vi "Digital Pattern Generation.vi"() -> ()   [LabVIEW 2020]
doc: "This example demonstrates how to acquire a continuous amount of digital data based off of a sample clock.\n\nSome hardware (e.g. M Series DAQ) must use an external sample clock for digital tasks. To view a complete list of available sample clock sources, consult the Device Routes table in Measurement and Automation Explorer.\n\nFor instructions on how to connect your signals to the DAQ device, refer to your device documentation."
uses:
  <vilib>/Utility/error.llb/DialogType.ctl
  <vilib>/DAQmx/read.llb/DAQmx Read (Digital Wfm 1Chan NSamp).vi
  <vilib>/DAQmx/create/channels.llb/DAQmx Create Channel (DI-Digital Input).vi
  <vilib>/Utility/file.llb/Read Delimited Spreadsheet (DBL).vi
  <vilib>/DAQmx/configure/timing.llb/DAQmx Timing (Sample Clock).vi
  <vilib>/DAQmx/miscellaneous.llb/DAQmx Fill In Error Info.vi
  <vilib>/Waveform/DWDTOps.llb/DWDT Digital to Analog.vi
  <vilib>/Analysis/polynomials.llb/Unique Numbers and Multiplicity (DBL).vi
  <vilib>/Analysis/NI_AALPro.lvlib
panel:
  in  "Crank or Cam":enum16{"Crank", "Cam"}(ring)
  out "Pass?":bool=TRUE
  out "Waveform Graph 2":waveform(dbl)(graph)={"t0"=timestamp(0 s since 1904-01-01), "dt"=0.0001, "Y"=array[40000 elements]}
  out "indices of samples equal to 1":i32[](array[numeric])
  out "number of samples equal to 1":i32=6448
  out "number of samples in each valley":i32[](array[numeric])=[140, 139, 140, 140, 140, 140, 140, 140, 140, 140, 139, 140, 140, 139, 140, 140, 139, 140, 140, 140, 140, 140, 140, 140, 140, 139, 140, 140, 139, 140, 140, 140, 140, 473, 140, 140, 140, 140, 139, 140, 140, 140, 140, 140, 140, 140, 140, 140, 140, 140, 140, 140, 140, 140, 140, 140, 140, 140, 140, 139, 140, 140, 140, 140, 140, 140, 140, 140, 139, 140, 140, 139, 140, 140, 139, 140, 140, 140, 140, 140, 140, 140, 140, 139, 140, 140, 139, 140, 140, 140, 140, 473, 140, 140, 140, 140, 139, 140, 140, 140, 140, 140, 140, 140, 140, 140, 140, 140, 140, 140, 140, 140, 140, 140, 140, 140, 140, 139, 140, 140, 140, 140, 140, 140, 140, 140, 139, 140, 140, 139, 140, 140, 139, 140, 140, 140, 140, 140, 140, 140, 140, 139, 140, 140, 139, 140, 140, 140, 140, 473, 140, 140, 140, 140, 139, 140, 140, 140, 140, 140, 140, 140, 140, 140, 140, 140, 140, 140, 140, 140, 140, 140, 140, 140, 140, 139, 140, 140, 140, 140, 140, 140, 140, 140, 139, 140, 140, 139, 140, 140, 139, 140, 140, 140, 140, 140, 140, 140, 140, 139, 140, 140, 139, 140, 140, 140, 140, 473, 140, 140, 140, 140, 139, 140, 140, 140, 140, 140, 140, 140, 140, 140, 140, 140, 140, 140, 140, 140, 140, 140, 140]
  out "number of valleys":i32=231
  out "number of valleys":i32=231
  out "number of samples in each valley":i32[](array[numeric])=[141, 140, 140, 140, 140, 140, 139, 140, 140, 139, 140, 140, 140, 140, 140, 140, 140, 140, 140, 140, 140, 139, 140, 140, 139, 140, 140, 140, 140, 140, 140, 140, 140, 140, 140, 140, 139, 140, 140, 140, 140, 140, 140, 140, 473, 140, 140, 140, 140, 140, 140, 140, 140, 140, 140, 140, 140, 140, 140, 140, 140, 140, 140, 140, 140, 140, 140, 140, 140, 140, 140, 140, 140, 140, 140, 140, 140, 140, 140, 140, 140, 140, 140, 140, 140, 140, 140, 140, 140, 140, 140, 140, 139, 140, 140, 140, 140, 140, 140, 140, 140, 140, 473, 140, 140, 139, 140, 140, 140, 140, 140, 140, 140, 140, 139, 140, 140, 139, 140, 140, 139, 140, 140, 140, 140, 140, 139, 140, 140, 139, 140, 140, 139, 140, 140, 139, 140, 140, 140, 140, 140, 139, 140, 140, 139, 140, 140, 139, 140, 140, 140, 140, 140, 140, 140, 140, 139, 140, 140, 139, 474, 140, 140, 140, 140, 140, 140, 140, 140, 139, 140, 140, 140, 140, 140, 140, 140, 140, 140, 140, 140, 140, 140, 140, 140, 140, 140, 140, 140, 140, 140, 140, 140, 140, 140, 140, 140, 140, 140, 140, 140, 140, 140, 140, 140, 140, 140, 140, 140, 140, 140, 140, 140, 140, 140, 140, 140, 140, 474, 140, 140, 140, 140, 140, 140, 139, 140, 140, 140, 140, 140]
  out "Waveform Graph":waveform(dbl)(graph)={"t0"=timestamp(3585136830.519799 s since 1904-01-01), "dt"=9.999999999999999e-05, "Y"=array[40000 elements], "attributes"=variant("NI_ChannelName"=variant(string "cDAQ1Mod1/port0/line0"), "NI_LineNames"=variant(string "cDAQ1Mod1/port0/line0"))}
  out "number of samples equal to 1":i32=6438
  out "indices of samples equal to 1":i32[](array[numeric])
  in  "Duration":i32=4
  in  "RPM":dbl=60.0
  in  "Sample Clock Source":tag="OnboardClock"
  in  "Line(s)":tag="cDAQ1Mod1/port0/line0"
  # "This test compares acquired data with reference data in terms of number of valleys, number of samples in each \nvalley, and number of samples equal to 1"
  # "Channel Settings"
  # "Acquired Data"
  # "Reference Data"
  # "Use line 0 for Crank and line 1 for Cam"
  # "Timing Settings"
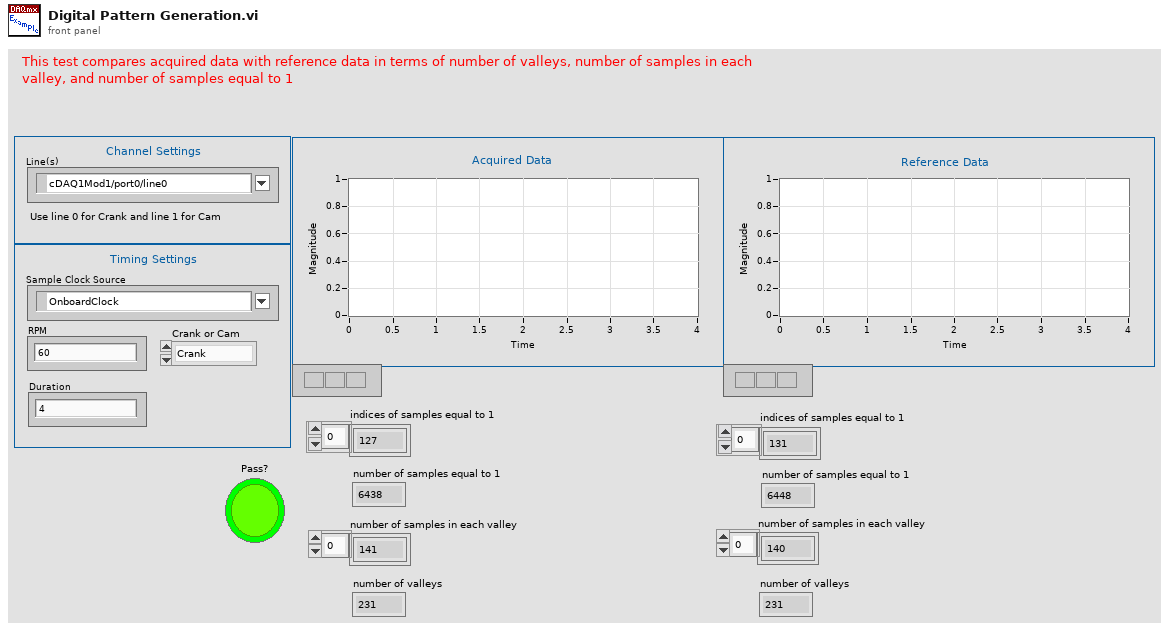
[diagram p1: front panel]
types:
  T1 = typedef "DialogType.ctl" = u16
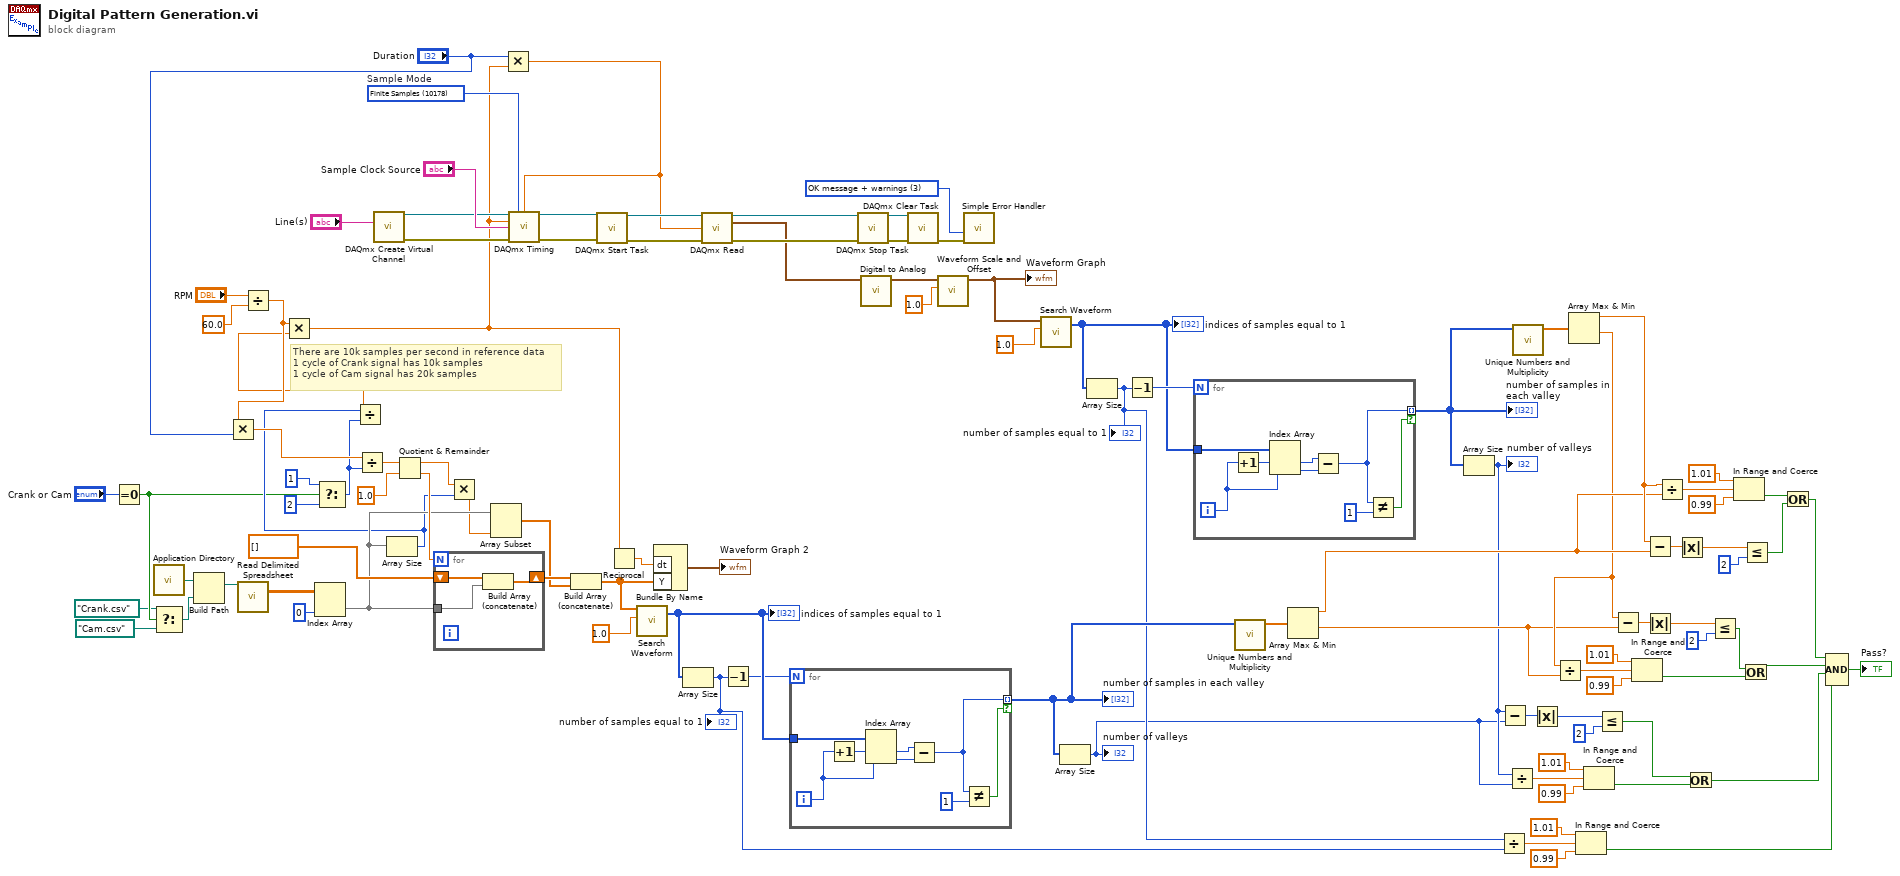
[diagram p0: block diagram]
diagram:
  w90 = T1 3 items=["no dialog", "OK message", "continue or stop message", "OK message + warnings", "continue/stop + warnings"] ("type of dialog (OK msg:1)")
  w100 = 10178 items=["Finite Samples"=10178, "Continuous Samples"=10123, "Hardware Timed Single Point"=12522]  # Sample Mode
  # "There are 10k samples per second in reference data\n1 cycle of Crank signal has 10k samples\n1 cycle of Cam signal has 20k samples"
  n1 = Equal To 0?(x="Crank or Cam") -> (x = 0?=w4:bool)
  n2 = call <vilib>:"Application Directory.vi"() -> ("Application Directory"=w6:path)
  n3 = Select(t=path "Crank.csv", s=w4, f=path "Cam.csv") -> (s? t:f=w1:path)
  n4 = Build Path(base path=w6, name or relative path=w1) -> (appended path=w5:path)
  n5 = call-poly <vilib>:"Read Delimited Spreadsheet.vi"("file path (dialog if empty)"=w5) -> ("all rows"=w57:dbl[][])  [unwired: 9 in, 5 out]
  n6 = Divide(x="RPM", y=60.0) -> (x/y=w49:dbl)
  n7 = Multiply(x=w49, y="Duration") -> (x*y=w48:dbl)
  n8 = Index Array(array=w57, index (col)=0 ("disabled index (col)")) -> (element=w39:dbl[])  [unwired: 1 in]
  n9 = Select(t=1, s=w4, f=2 ("y")) -> (s? t:f=w33:i32)
  n10 = Divide(x=w48, y=w33) -> (x/y=w42:dbl)
  n11 = call-poly <vilib>:"DAQmx Create Virtual Channel.vi"("lines"="Line(s)") -> ("task out"=w98:refnum<k21>, "error out"=w97:errorcluster)  [unwired: 13 in]
  n12 = Array Size(array=w39) -> (size(s)=w34:i32)
  n13 = Divide(x=w34, y=w33) -> (x/y=w32:dbl)
  n14 = Multiply(x=w49, y=w32) -> (x*y=w44:dbl)
  n15 = Quotient & Remainder(x=w42, y=1.0) -> (x-y*floor(x/y)=w38:dbl, floor(x/y)=w40:dbl)
  n16 = for {
    N: w40 -> [_]
    shift-right: [w103] -> w36
    shift-left: dbl[] [] -> [w105]
    tunnel: w39 -> [w104]
    n17 = Build Array (concatenate)(w105, w104) -> (w103:dbl[])
  }
  n18 = Multiply(x=w38, y=w34) -> (x*y=w37:dbl)
  n19 = Array Subset(array=w39, length=w37) -> (w35:dbl[])  [unwired: 1 in]
  n20 = Multiply(x="Duration", y=w44) -> (x*y=w53:dbl)
  n21 = call-poly <vilib>:"DAQmx Timing.vi"("task/channels in"=w98, "sample mode"=w100, "samples per channel"=w53, "rate"=w44, "source"="Sample Clock Source", "error in"=w97) -> ("task out"=w89:refnum<k21>, "error out"=w88:errorcluster)  [unwired: 8 in]
  n22 = Build Array (concatenate)(w36, w35) -> (w31:dbl[])
  n23 = call <vilib>:"DAQmx Start Task.vi"("task/channels in"=w89, "error in"=w88) -> ("task out"=w95:refnum<k21>, "error out"=w96:errorcluster)  [unwired: 12 in]
  n24 = Reciprocal(x=w44) -> (1/x=w43:dbl)
  n25 = call <vilib>:"Search Waveform.vi"("value"=1.0, "waveform in"=w31) -> ("indices of fits"=w82:i32[])  [unwired: 4 in, 5 out]
  "indices of samples equal to 1" <- w82
  n26 = Bundle By Name("dt"=w43, "Y"=w31) -> (→"Waveform Graph 2":waveform(dbl))  [unwired: 1 in]
  n27 = Array Size(array=w82) -> (size(s)=w65:i32)
  "number of samples equal to 1" <- w65
  n28 = call-poly <vilib>:"DAQmx Read.vi"("task/channels in"=w95, "number of samples per channel"=w53, "error in"=w96) -> ("task out"=w92:refnum<k21>, "data"=w59:digitalwaveform, "error out"=w91:errorcluster)  [unwired: 10 in]
  n29 = Decrement(x=w65) -> (x-1=w81:i32)
  n30 = for {
    N: w81 -> [_]
    tunnel: w82 -> [w113]
    tunnel: [w107] -> w79 mode=indexing if=w106
    i -> [w108]
    n31 = Increment(x=w108) -> (x+1=w112:i32)
    n32 = Index Array(array=w113, index #1=w112, index #2=w108) -> (element #1=w110:i32, element #2=w111:i32)
    n33 = Subtract(x=w110, y=w111) -> (x-y=w107:i32)
    n34 = Not Equal?(x=w107, y=1) -> (x != y?=w106:bool)
  }
  "number of samples in each valley" <- w79
  n35 = call <vilib>:"DAQmx Stop Task.vi"("task/channels in"=w92, "error in"=w91) -> ("task out"=w94:refnum<k21>, "error out"=w93:errorcluster)  [unwired: 12 in]
  n36 = call-poly <vilib>:"Digital to Analog.vi"("digital waveform"=w59) -> ("analog waveform"=w87:waveform(dbl))  [unwired: 7 in, 3 out]
  n37 = call <vilib>:"DAQmx Clear Task.vi"("task in"=w94, "error in"=w93) -> ("error out"=w102:errorcluster)  [unwired: 13 in]
  n38 = call <vilib>:"Waveform Scale and Offset.vi"("offset"=1.0, "waveform in"=w87) -> ("waveform out"=w58:waveform(dbl))  [unwired: 8 in, 1 out]
  "Waveform Graph" <- w58
  n39 = call <vilib>:"Simple Error Handler.vi"("type of dialog (OK msg:1)"=w90, "error in (no error)"=w102) -> ()  [unwired: 3 in, 5 out]
  n40 = call <vilib>:"Search Waveform.vi"("value"=1.0, "waveform in"=w58) -> ("indices of fits"=w83:i32[])  [unwired: 4 in, 5 out]
  "indices of samples equal to 1" <- w83
  n41 = Array Size(array=w79) -> (size(s)=w10:i32)
  "number of valleys" <- w10
  n42 = Array Size(array=w83) -> (size(s)=w66:i32)
  "number of samples equal to 1" <- w66
  n43 = Decrement(x=w66) -> (x-1=w84:i32)
  n44 = for {
    N: w84 -> [_]
    tunnel: w83 -> [w121]
    tunnel: [w115] -> w78 mode=indexing if=w114
    i -> [w116]
    n45 = Increment(x=w116) -> (x+1=w120:i32)
    n46 = Index Array(array=w121, index #1=w120, index #2=w116) -> (element #1=w118:i32, element #2=w119:i32)
    n47 = Subtract(x=w118, y=w119) -> (x-y=w115:i32)
    n48 = Not Equal?(x=w115, y=1) -> (x != y?=w114:bool)
  }
  "number of samples in each valley" <- w78
  n49 = call-poly <vilib>:"Unique Numbers and Multiplicity.vi"("Numbers"=w79) -> ("Unique Numbers"=w73:dbl[])  [unwired: 8 in, 2 out]
  n50 = Array Max & Min(array=w73) -> (max value=w26:dbl, min value=w18:dbl)  [unwired: 2 out]
  n51 = Array Size(array=w78) -> (size(s)=w11:i32)
  "number of valleys" <- w11
  n52 = Divide(x=w66, y=w65) -> (x/y=w64:dbl)
  n53 = Subtract(x=w11, y=w10) -> (x-y=w77:i32)
  n54 = Divide(x=w11, y=w10) -> (x/y=w12:dbl)
  n55 = call-poly <vilib>:"Unique Numbers and Multiplicity.vi"("Numbers"=w78) -> ("Unique Numbers"=w74:dbl[])  [unwired: 8 in, 2 out]
  n56 = Absolute Value(x=w77) -> (abs(x)=w76:i32)
  n57 = Array Max & Min(array=w74) -> (max value=w27:dbl, min value=w19:dbl)  [unwired: 2 out]
  n58 = Divide(x=w19, y=w18) -> (x/y=w22:dbl)
  n59 = In Range and Coerce(upper limit=1.01, x=w64, lower limit=0.99) -> (In Range?=w61:bool)  [unwired: 1 out]
  n60 = In Range and Coerce(upper limit=1.01, x=w12, lower limit=0.99) -> (In Range?=w9:bool)  [unwired: 1 out]
  n61 = Less Or Equal?(x=w76, y=2) -> (x <= y?=w8:bool)
  n62 = Subtract(x=w19, y=w18) -> (x-y=w70:dbl)
  n63 = In Range and Coerce(upper limit=1.01, x=w22, lower limit=0.99) -> (In Range?=w17:bool)  [unwired: 1 out]
  n64 = Subtract(x=w27, y=w26) -> (x-y=w69:dbl)
  n65 = Absolute Value(x=w70) -> (abs(x)=w71:dbl)
  n66 = Divide(x=w27, y=w26) -> (x/y=w28:dbl)
  n67 = Absolute Value(x=w69) -> (abs(x)=w68:dbl)
  n68 = Or(x=w8, y=w9) -> (x .or. y?=w7:bool)
  n69 = Less Or Equal?(x=w71, y=2) -> (x <= y?=w16:bool)
  n70 = In Range and Coerce(upper limit=1.01, x=w28, lower limit=0.99) -> (In Range?=w25:bool)  [unwired: 1 out]
  n71 = Or(x=w16, y=w17) -> (x .or. y?=w15:bool)
  n72 = Less Or Equal?(x=w68, y=2) -> (x <= y?=w24:bool)
  n73 = Or(x=w25, y=w24) -> (x .or. y?=w23:bool)
  n74 = Compound Arithmetic op=AND(w23, w15, w7, w61) -> (→"Pass?":bool)
